vi "KTRL_ENCODE.vi"(1 "Argumento":string, 2 "Etiqueta":string) -> (0 "Salida":string)   [LabVIEW 2017]
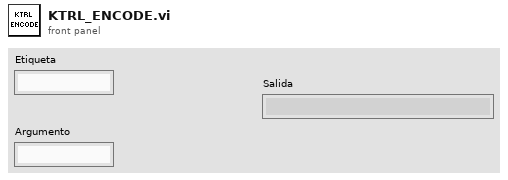
[diagram p1: front panel]
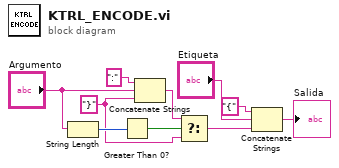
[diagram p0: block diagram]
diagram:
  w2 = "}"
  n1 = String Length(string="Argumento") -> (length=w10:i32)
  n2 = Greater Than 0?(x=w10) -> (x > 0?=w7:bool)
  n3 = Concatenate Strings(":", "Argumento", w2) -> (w1:string)
  n4 = Select(t=w1, s=w7, f=w2) -> (s? t:f=w6:string)
  n5 = Concatenate Strings("{", "Etiqueta", w6) -> (→"Salida":string)
